vi "UMLEditor PrintDialog.vi"(2 "Permissions":cluster{"SaveToFile":bool}, 5 "error in (no error)":errorcluster={"status"=FALSE, "code"=200021, "source"="DAQmx Write (Analog DBL 1Chan 1Samp).vi"}) -> (15 "PrinterInfo":T1={"PrinterName"="\\\\PLUTO\\Canon GP225", "Copies"=1, "PrintToFile"=FALSE, "orientation"=0, "PaperSize"=1} {"PaperSize" items=["PaperLetter"=1, "PaperLetterSmall"=2, "PaperTabloid"=3, "PaperLedger"=4, "PaperLegal"=5, "PaperStatement"=6, "PaperExecutive"=7, "PaperA3"=8, "PaperA4"=9, "PaperA4Small"=10, "PaperA5"=11, "PaperB4"=12, "PaperB5"=13, "PaperFolio"=14, "PaperQuarto"=15, "Paper10x14"=16, "Paper11x17"=17, "PaperNote"=18, "PaperEnvelop9"=19, "PaperEnvelop10"=20, "PaperEnvelop11"=21, "PaperEnvelop12"=22, "PaperEnvelop14"=23, "PaperCSheet"=24, "PaperDSheet"=25, "PaperESheet"=26, "PaperEnvelopDL"=27, "PaperEnvelopC5"=28, "PaperEnvelopC3"=29, "PaperEnvelopC4"=30, "PaperEnvelopC6"=31, "PaperEnvelopC65"=32, "PaperEnvelopB4"=33, "PaperEnvelopB5"=34, "PaperEnvelopB6"=35, "PaperEnvelopItaly"=36, "PaperEnvelopMonarch"=37, "PaperEnvelopPersonal"=38, "PaperFanFoldUS"=39, "PaperFanFoldStandardGerman"=40, "PaperFanFoldLegalGerman"=41, "PaperISOB4"=42, "PaperJapanesePostcard"=43, "Paper9X11"=44, "Paper10X11"=45, "Paper15X11"=46, "PaperEnvelopInvite"=47, "PaperLetterExtra"=50, "PaperLegalExtra"=51, "PaperTabloidExtra"=52, "PaperA4Extra"=53, "PaperLetterTransverse"=54, "PaperA4Transverse"=55, "PaperLetterExtraTransverse"=56, "PaperAPlus"=57, "PaperBPlus"=58, "PaperLetterPlus"=59, "PaperA4Plus"=60, "PaperA5Transverse"=61, "PaperB5Transverse"=62, "PaperA3Extra"=63, "PaperA5Extra"=64, "PaperB5Extra"=65, "PaperA2"=66, "PaperA3Transverse"=67, "PaperA3ExtraTransverse"=68]; "orientation" items=["portrait", "landscape"]}, 16 "Cancelled":bool, 19 "error out":errorcluster={"status"=FALSE, "code"=200021, "source"="DAQmx Write (Analog DBL 1Chan 1Samp).vi"})   [LabVIEW 2016]
uses:
  <resource>/Framework/Providers/Open_GDS/UML/UMLEditor/UMLEditor PrinterSettings.ctl
  Instance           1 29Saved   UMLEditor PrintDialog .vi
  <vilib>/Utility/NIReport.llb/NI_ReportGenerationCore.lvlib
panel:
  in  "Name:":u16(ring) items=["Microsoft Office Document Image Writer", "Lexmark Z53 Color Jetprinter", "HP Business Inkjet 2200/2250 (HPA)", "Auto DeskJet 990cxi on PLUTO", "Auto Canon GP225 on PLUTO", "\\\\PLUTO\\DeskJet 990cxi"]
  in  "Landscape":bool
  in  "Portrait":bool=TRUE
  in  "Number of copies:":i32=1 min=1
  in  "ToFile":bool
  in  "Cancel":bool
  in  "Ok":bool
  in  "Locals":T2
  # "Configure your printer"
  # "Select printer and configure the output"
  # "Printer"
  # "Paper Orientation"
  # "Copies"
  # "3"
  # "2"
  # "1"
  # "Name:"
  # "A"
  # "A"
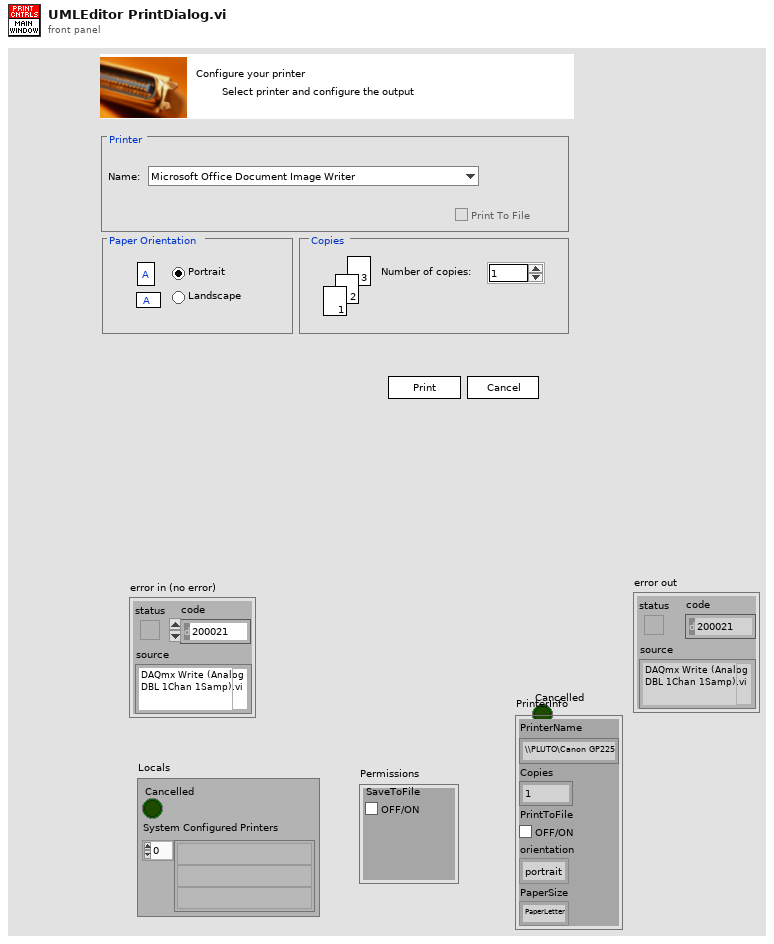
[diagram p1: front panel]
types:
  T1 = typedef "UMLEditor PrinterSettings.ctl" = cluster{"PrinterName":string, "Copies":i32, "PrintToFile":bool, "orientation":u16, "PaperSize":i32}
  T2 = cluster{"Cancelled":bool, "System Configured Printers":string[]}
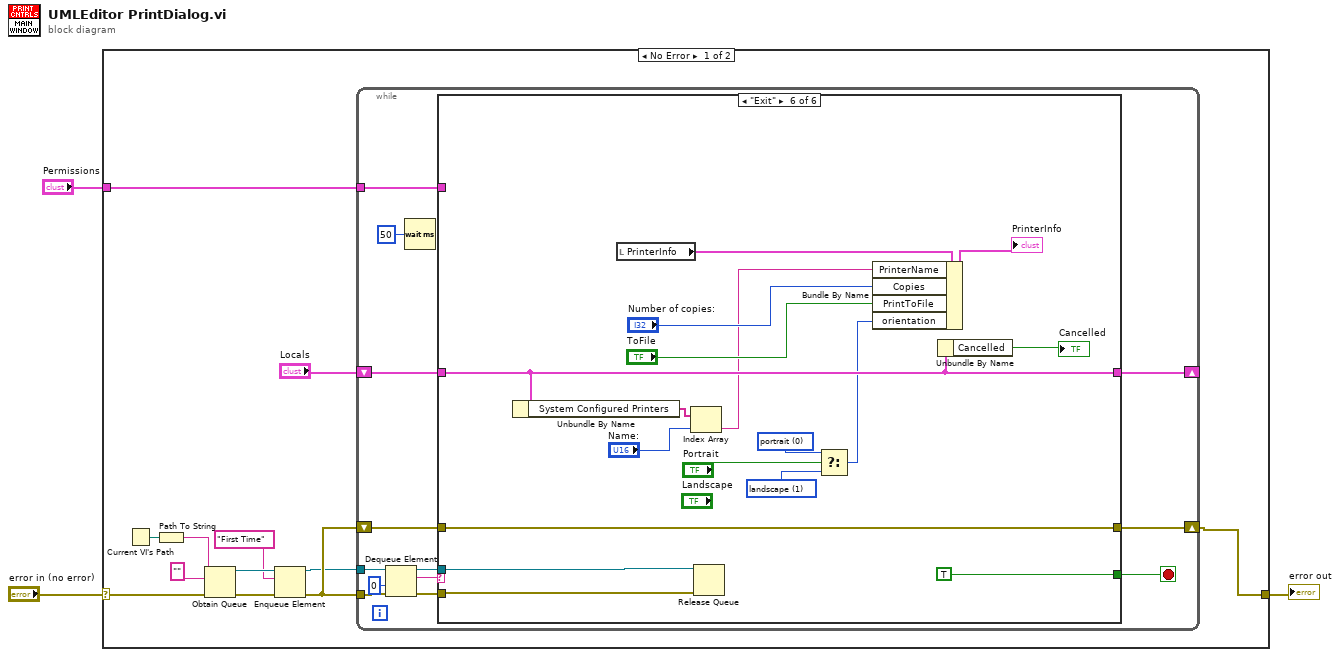
[diagram p0: block diagram]
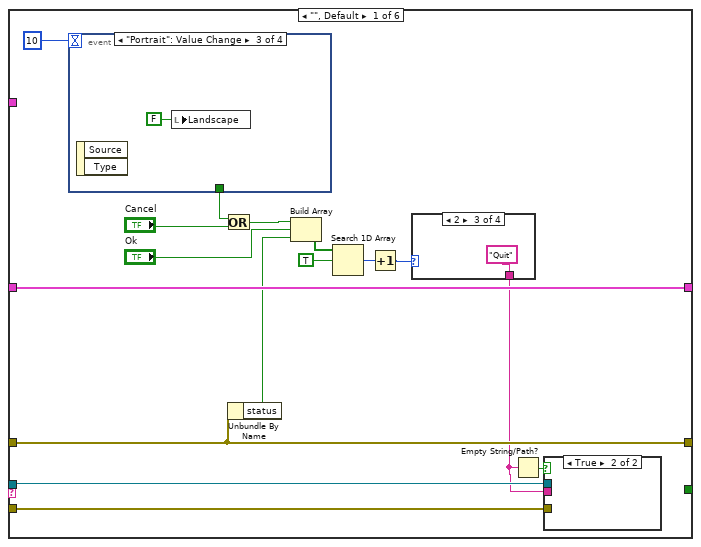
[diagram p2: hidden frame]
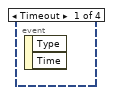
[diagram p3: hidden frame]
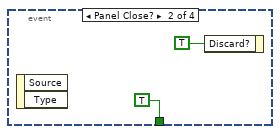
[diagram p4: hidden frame]
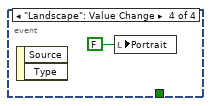
[diagram p5: hidden frame]
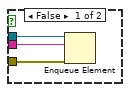
[diagram p6: hidden frame]
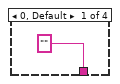
[diagram p7: hidden frame]
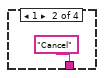
[diagram p8: hidden frame]
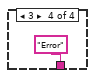
[diagram p9: hidden frame]
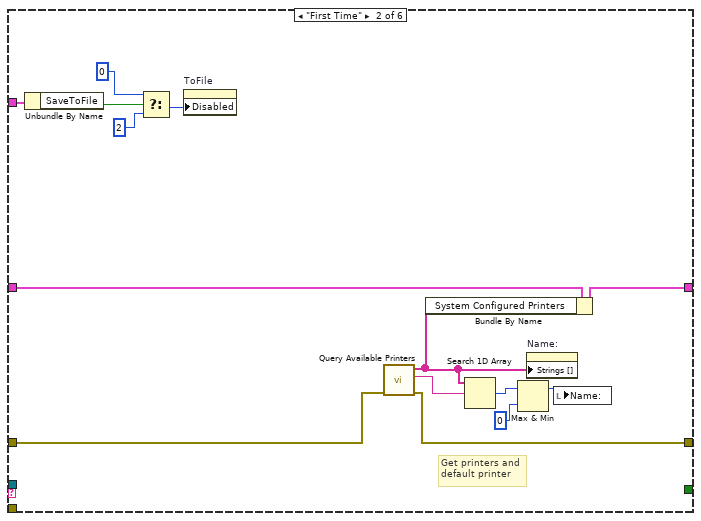
[diagram p10: hidden frame]
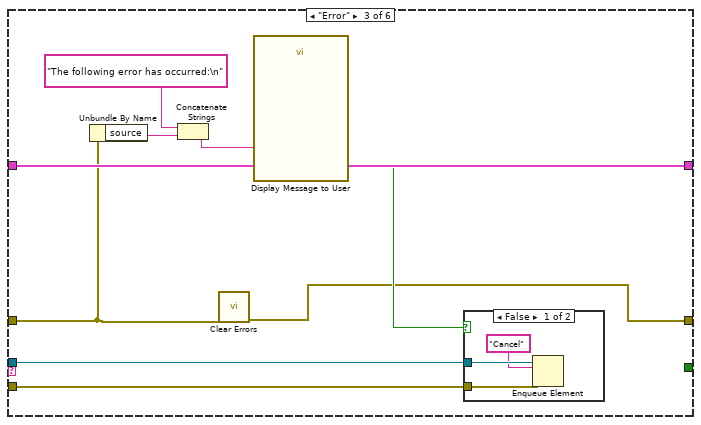
[diagram p11: hidden frame]
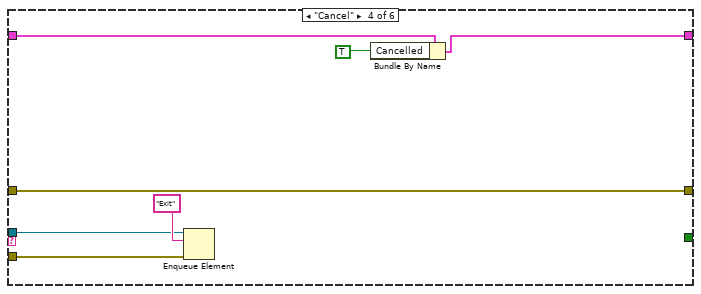
[diagram p13: hidden frame]
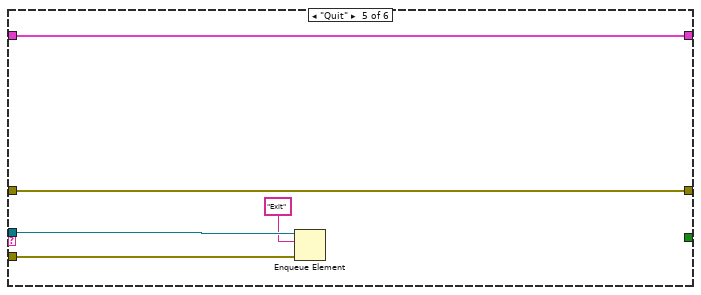
[diagram p14: hidden frame]
diagram:
  n1 = case shown="No Error" "error in (no error)" {
    selector: "error in (no error)" -> [w15 w111]
    tunnel: [w6 w111] -> w2
    tunnel: "Permissions" -> [w4 _]
    frame No Error {
      n2 = Current VI's Path() -> (path=w14:path)
      n3 = Path To String(path=w14) -> (string=w13:string)
      n4 = Obtain Queue(name (unnamed)=w13, element data type="", error in (no error)=w15) -> (queue out=w10:refnum<queue>, error out=w11:errorcluster)  [unwired: 2 in, 1 out]
      n5 = Enqueue Element(queue=w10, element="First Time", error in (no error)=w11) -> (queue out=w7:refnum<queue>, error out=w8:errorcluster)  [unwired: 2 out]
      n6 = while {
        shift-right: [w22] -> w6
        shift-left: w8 -> [w23]
        tunnel: w8 -> [w28]
        tunnel: w7 -> [w27]
        shift-right: [w19] -> _
        shift-left: "Locals" -> [w20]
        tunnel: w4 -> [w16]
        stop <- w21 stop-if-true
        n7 = Dequeue Element(queue=w27, timeout in ms (-1)=0, error in (no error)=w28) -> (queue out=w24:refnum<queue>, element=w25:string, error out=w26:errorcluster)  [unwired: 1 out]
        n8 = Wait (ms)(milliseconds to wait=u32 50) -> ()  [unwired: 1 out]
        n9 = case shown="\"Exit\"" w25 {
          tunnel: w26 -> [w38 _ w73 w86 w91 w107]
          tunnel: w24 -> [w37 _ w72 w85 w90 w108]
          tunnel: w23 -> [w43 w68 w71 w88 w92 w109]
          tunnel: [w43 w67 w70 w88 w92 w109] -> w22
          tunnel: [_ _ _ _ _ TRUE] -> w21
          tunnel: w20 -> [w44 w66 w78 w84 w93 w101]
          tunnel: [w44 w65 w78 w83 w93 w101] -> w19
          tunnel: w16 -> [_ w60 _ _ _ _]
          frame "", Default {
            n10 = event shown="[2] \"Portrait\": Value Change" {
              selector: _ -> [_ _ _ _]
              dyn-events: _ -> [_ _ _ _]
              timeout: 10 -> [_ _ _ _]
              tunnel: [_ TRUE ("Discard?") _ _] -> w32
              event Timeout {
                n11 = event-data() -> ()  [unwired: 3 out]
              }
              event Panel Close? {
                n12 = event-data() -> ()  [unwired: 3 out]
                n13 = event-data("Discard?"=TRUE) -> ()  [unwired: 1 in, 1 out]
              }
              event "Portrait": Value Change {
                n14 = event-data() -> ()  [unwired: 3 out]
                n15 = local write "Landscape"(FALSE ("Landscape")) -> ()
              }
              event "Landscape": Value Change {
                n16 = event-data() -> ()  [unwired: 3 out]
                n17 = local write "Portrait"(FALSE ("Portrait")) -> ()
              }
            }
            n18 = Or(x=w32, y="Cancel") -> (x .or. y?=w33:bool)
            n19 = Unbundle By Name(w43) -> ("status"=w29:bool)
            n20 = Build Array(w33, "Ok", w29) -> (w42:bool[])
            n21 = Search 1D Array(1D array=w42, element=TRUE) -> (index of element=w40:i32)  [unwired: 1 out]
            n22 = Increment(x=w40) -> (x+1=w39:i32)
            n23 = case shown="2" w39 {
              tunnel: ["" "Cancel" "Quit" "Error"] -> w35
              frame 0, Default {
              }
              frame 1 {
              }
              frame 2 {
              }
              frame 3 {
              }
            }
            n24 = Empty String/Path?(string/path=w35) -> (empty?=w36:bool)
            n25 = case shown="True" w36 {
              tunnel: w38 -> [w51 _]
              tunnel: w37 -> [w50 _]
              tunnel: w35 -> [w49 _]
              frame False {
                n26 = Enqueue Element(queue=w50, element=w49, error in (no error)=w51) -> ()  [unwired: 4 out]
              }
              frame True {
              }
            }
          }
          frame "First Time" {
            # "Get printers and\ndefault printer"
            n27 = Unbundle By Name(w60) -> ("SaveToFile"=w59:bool)
            n28 = Select(t=u8 0, s=w59, f=u8 2) -> (s? t:f=w57:u8)
            n29 = property on="ToFile" class="Bool (strict)"("Disabled"=w57) -> ()  [unwired: 2 in, 2 out]
            n30 = call <vilib>:"Query Available Printers.vi"("error in (no error)"=w68) -> ("error out"=w67:errorcluster, "default printer"=w69:string, "system configured printers"=w64:string[])  [unwired: 8 out]
            n31 = Bundle By Name(cluster=w66, "System Configured Printers"=w64) -> (w65:T2)
            n32 = Search 1D Array(1D array=w64, element=w69) -> (index of element=w63:i32)  [unwired: 1 out]
            n33 = Max & Min(x=w63, y=0) -> (max(x,y)=w61:i32)  [unwired: 1 out]
            n34 = property on="Name:" class="Ring (strict)"("Strings []"=w64) -> ()  [unwired: 2 in, 2 out]
            n35 = local write "Name:"(w61) -> ()
          }
          frame "Error" {
            n36 = Unbundle By Name(w71) -> ("source"=w76:string)
            n37 = Concatenate Strings("The following error has occurred:\n" ("string"), w76) -> (w75:string)
            n38 = call <vilib>:"Clear Errors.vi"("error in (no error)"=w71) -> ("error out"=w70:errorcluster)  [unwired: 1 in, 5 out]
            n39 = call "Display Message to User"("Message"=w75) -> ("Ignore"=w74:bool)  [unwired: 2 in, 8 out]
            n40 = case shown="False" w74 {
              tunnel: w73 -> [w80 _]
              tunnel: w72 -> [w81 _]
              frame False {
                n41 = Enqueue Element(queue=w81, element="Cancel", error in (no error)=w80) -> ()  [unwired: 4 out]
              }
              frame True {
              }
            }
          }
          frame "Cancel" {
            n42 = Enqueue Element(queue=w85, element="Exit", error in (no error)=w86) -> ()  [unwired: 4 out]
            n43 = Bundle By Name(cluster=w84, "Cancelled"=TRUE) -> (w83:T2)
          }
          frame "Quit" {
            n44 = Enqueue Element(queue=w90, element="Exit", error in (no error)=w91) -> ()  [unwired: 4 out]
          }
          frame "Exit" {
            w94 = u16 1 items=["portrait", "landscape"] ("orientation (portrait)")
            w95 = u16 0 items=["portrait", "landscape"] ("orientation (portrait)")
            n45 = Unbundle By Name(w101) -> ("System Configured Printers"=w100:string[])
            n46 = local read "PrinterInfo"() -> (w106:T1)
            n47 = Index Array(array=w100, index="Name:") -> (element=w98:string)
            n48 = Release Queue(queue=w108, error in (no error)=w107) -> ()  [unwired: 4 out]
            n49 = Select(t=w95, s="Portrait", f=w94) -> (s? t:f=w96:u16)
            n50 = Bundle By Name(cluster=w106, "PrinterName"=w98, "Copies"="Number of copies:", "PrintToFile"="ToFile", "orientation"=w96) -> (→"PrinterInfo":T1)
            n51 = Unbundle By Name(w101) -> ("Cancelled"=→"Cancelled":bool)
          }
        }
      }
    }
    frame Error {
    }
  }
  "error out" <- w2
